vi "Get Current Operating Mode.vi"(8 "error in (no error)":errorcluster, 11 "VISA resource name":refnum<visa-resource-name>) -> (0 "error out":errorcluster, 2 "Operating Mode":i32(ring) items=["Weighing", "Parts Counting", "Deviations", "Dosing", "Animals Weighing", "Formulas", "Density", "Density of Solid Bodies", "Density of Liquids", "Peak Hold", "Totalizing", "Checkweighin", "Statistics", "Pipettes Calibration", "Differential Weighing", "Statistical Quality Control (SQC)", "Product Inspection", "Weight Control (Tableting)", "Drying", "Comparator", "Weighbridge"], 3 "VISA resource name out":refnum<visa-resource-name>)   [LabVIEW 2017, in "RadWag balances and scales.lvlib"]
doc: "Gets balance current operating mode. Operating mode can be changed via \"Set Operating Mode\" VI, as well as from balance keyboard."
uses:
  <instrlib>/Radwag Balances and Scales/Public/RadWag Continuous Read Folder/RadWag balances and scales.lvlib
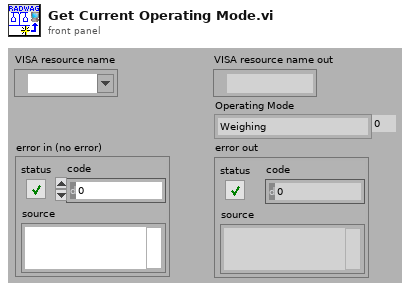
[diagram p1: front panel]
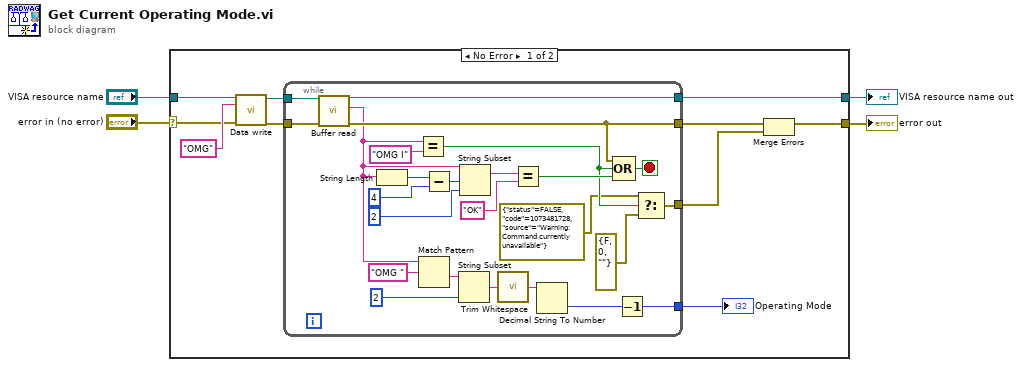
[diagram p0: block diagram]
diagram:
  n1 = case shown="No Error" "error in (no error)" {
    selector: "error in (no error)" -> [w9 w40]
    tunnel: "VISA resource name" -> [w14 w41]
    tunnel: [w11 w41] -> w3
    tunnel: [w7 w40] -> w2
    frame No Error {
      n2 = call <instrlib>:"Data write.vi"("error in (no error)"=w9, "ID"="OMG", "VISA resource name"=w14) -> ("error out"=w12:errorcluster, "VISA resource name out"=w13:refnum<visa-resource-name>)  [unwired: 7 in]
      n3 = while {
        tunnel: w13 -> [w38]
        tunnel: w12 -> [w37]
        tunnel: [w36] -> w11
        tunnel: [w25] -> w8
        tunnel: [w15] -> w5
        tunnel: [w17] -> w6
        stop <- w39 stop-if-true
        n4 = call <instrlib>:"Buffer read.vi"("error in (no error)"=w37, "VISA resource name"=w38) -> ("error out"=w25:errorcluster, "Received String"=w21:string, "VISA resource name out"=w36:refnum<visa-resource-name>)  [unwired: 7 in]
        n5 = String Length(string=w21) -> (length=w32:i32)
        n6 = Equal?(x=w21, y="OMG I" ("x")) -> (x = y?=w19:bool)
        n7 = Match Pattern(string=w21, regular expression="OMG ") -> (after substring=w29:string)  [unwired: 1 in, 3 out]
        n8 = Subtract(x=w32, y=4) -> (x-y=w33:i32)
        n9 = String Subset(string=w29, length (rest)=2 ("length (rest)")) -> (substring=w27:string)  [unwired: 1 in]
        n10 = String Subset(string=w21, offset (0)=w33, length (rest)=2 ("length (rest)")) -> (substring=w23:string)
        n11 = call <vilib>:"Trim Whitespace.vi"("string"=w27) -> ("trimmed string"=w26:string)  [unwired: 1 in]
        n12 = Equal?(x=w23, y="OK") -> (x = y?=w20:bool)
        n13 = Decimal String To Number(string=w26) -> (number=w24:i32)  [unwired: 2 in, 1 out]
        n14 = Compound Arithmetic op=OR(w25, w19, w20) -> (w39:bool)
        n15 = Decrement(x=w24) -> (x-1=w15:i32)
        n16 = Select(t=errorcluster {"status"=FALSE, "code"=1073481728, "source"="Warning: Command currently unavailable"}, s=w19, f=errorcluster {"status"=FALSE, "code"=0, "source"=""} ("t")) -> (s? t:f=w17:errorcluster)
      }
      "Operating Mode" <- w5
      n17 = Merge Errors(w8, w6) -> (w7:errorcluster)
    }
    frame Error {
    }
  }
  "VISA resource name out" <- w3
  "error out" <- w2
